vi "GetParameterInfo.vi"(7 "Camera Parameter":T2, 8 "error in (no error)":errorcluster, 11 "Stream in":refnum<class "Stream.lvclass">) -> (0 "error out":errorcluster, 2 "Info":T1, 3 "Stream":refnum<class "Stream.lvclass">)   [LabVIEW 2020, in "capture.lvlib" / "Stream.lvclass"]
doc: "GetParameterInfo."
uses:
  Stream.lvclass
  Camera Parameters.ctl
  Camera Parameter Information.ctl
  Stream.lvclass/Stream.ctl
  common/common.lvlib
  common/bin/gartoolkit_32-1.dll
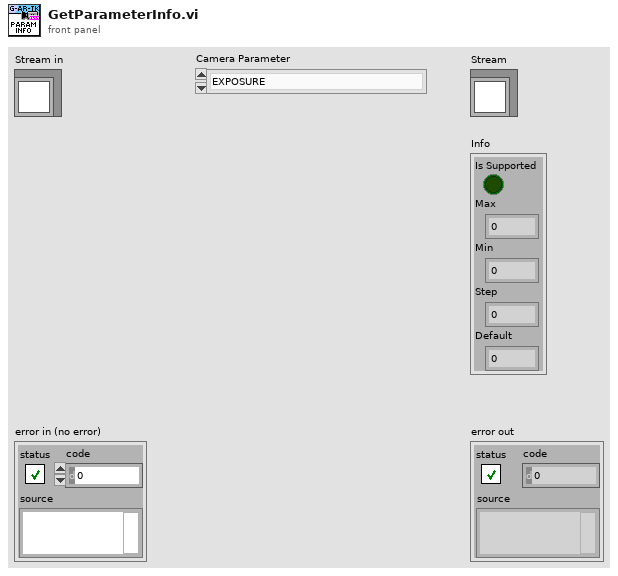
[diagram p1: front panel]
types:
  T1 = typedef "capture.lvlib/Stream.lvclass/Camera Parameter Information.ctl" = cluster{"Is Supported":bool, "Max":i32, "Min":i32, "Step":i32, "Default":i32}
  T2 = typedef "capture.lvlib/Stream.lvclass/Camera Parameters.ctl" = enum8{"EXPOSURE", "FOCUS", "ZOOM", "GAIN", "WHITE_BALANCE_TEMPERATURE", "BRIGHTNESS", "CONTRAST", "SATURATION", "GAMMA", "HUE", "SHARPNESS", "BACKLIGHT_COMPENSATION", "POWER_LINE_FREQUENCY"}
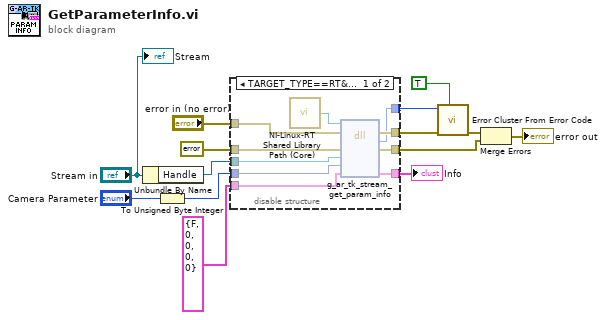
[diagram p0: block diagram]
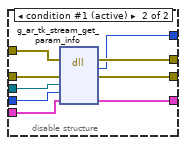
[diagram p2: hidden frame]
diagram:
  n1 = Unbundle By Name("Stream in") -> ("Handle"=w8:refnum<data-value>)
  n2 = To Unsigned Byte Integer(number="Camera Parameter") -> (unsigned 8bit integer=w7:u8)
  n3 = disable-structure shown="TARGET_TYPE==RT&&OS==Linux" {
    disable-tunnel: "error in (no error)" -> [w24 w33]
    disable-tunnel: errorcluster {"status"=FALSE, "code"=0, "source"=""} ("error constant") -> [w23 w32]
    disable-tunnel: w8 -> [w22 w31]
    disable-tunnel: w7 -> [w21 w30]
    disable-tunnel: T1 {"Is Supported"=FALSE, "Max"=0, "Min"=0, "Step"=0, "Default"=0} ("Camera Parameter Information") -> [w20 w29]
    disable-tunnel: [w19 w28] -> w5
    disable-tunnel: [w18 w27] -> w4
    disable-tunnel: [w17 w26] -> w3
    disable-tunnel: [w16 w25] -> w2
    frame condition #0 {
      n4 = call "NI-Linux-RT Shared Library Path (Core).vi"() -> ("Path"=w15:path)
      n5 = dll-call lib="?" fn="g_ar_tk_stream_get_param_info" ("g_ar_toolkit.*.*:g_ar_tk_stream_capture_next")(path in=w15, error in=w24, "error_cluster"=w23, "EDVR_strm"=w22, "parameter"=w21, "info"=w20) -> (error out=w19:errorcluster, w18:i32, "error_cluster"=w17:errorcluster, "info"=w16:T1)  [unwired: 3 in, 1 out]
    }
    frame condition #1 (active) {
      n6 = dll-call lib="C:/serenial/lib/g-augmented-reality-toolkit/LabVIEW/common/bin/gartoolkit_*-1.*" fn="g_ar_tk_stream_get_param_info" ("g_ar_toolkit.*.*:g_ar_tk_stream_capture_next")(error in=w33, "error_cluster"=w32, "EDVR_strm"=w31, "parameter"=w30, "info"=w29) -> (error out=w28:errorcluster, w27:i32, "error_cluster"=w26:errorcluster, "info"=w25:T1)  [unwired: 4 in, 1 out]
    }
  }
  "Info" <- w2
  n7 = call <vilib>:"Error Cluster From Error Code.vi"("show call chain? (False)"=TRUE, "error in (no error)"=w5, "error code (0)"=w4) -> ("error out"=w12:errorcluster)  [unwired: 6 in]
  n8 = Merge Errors(w12, w3) -> (→"error out":errorcluster)
  "Stream" <- "Stream in"
